vi "Check if Adjacent.vi"(8 "error in (no error)":errorcluster, 9 "Symbol.lvclass":refnum<class "Symbol.lvclass">, 10 "Number.lvclass":refnum<class "Number.lvclass">) -> (0 "error out":errorcluster, 2 "Is Adjacent?":bool)   [LabVIEW 2020, in "Schema Parser.lvclass"]
uses:
  Schema Parser.lvclass
  Number/Number.lvclass
  Symbol/Symbol.lvclass
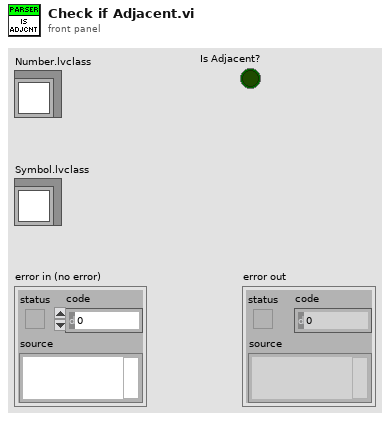
[diagram p1: front panel]
types:
  T1 = typedef "Symbol.lvclass/Coordinate.ctl" = cluster{"Col":i32, "Row":i32}
  T2 = typedef "Number.lvclass/Coordinate.ctl" = cluster{"Col":i32, "Row":i32}
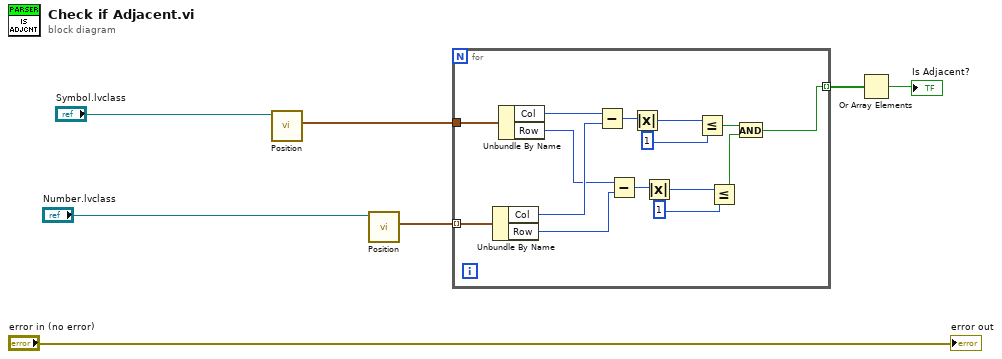
[diagram p0: block diagram]
diagram:
  n1 = call "Position.vi"("Number in"="Symbol.lvclass") -> ("Position"=w3:T1)  [unwired: 8 in, 2 out]
  n2 = call "Position.vi"("Number in"="Number.lvclass") -> ("Position"=w4:T2[])  [unwired: 8 in, 2 out]
  n3 = for {
    tunnel: w4 -> [w22] mode=indexing
    tunnel: w3 -> [w21]
    tunnel: [w9] -> w1 mode=indexing
    n4 = Unbundle By Name(w22) -> ("Col"=w19:i32, "Row"=w10:i32)
    n5 = Unbundle By Name(w21) -> ("Col"=w20:i32, "Row"=w11:i32)
    n6 = Subtract(x=w20, y=w19) -> (x-y=w18:i32)
    n7 = Subtract(x=w11, y=w10) -> (x-y=w12:i32)
    n8 = Absolute Value(x=w18) -> (abs(x)=w17:i32)
    n9 = Absolute Value(x=w12) -> (abs(x)=w13:i32)
    n10 = Less Or Equal?(x=w17, y=1) -> (x <= y?=w15:bool)
    n11 = Less Or Equal?(x=w13, y=1) -> (x <= y?=w8:bool)
    n12 = And(x=w15, y=w8) -> (x .and. y?=w9:bool)
  }
  n13 = Or Array Elements(Boolean array=w1) -> (logical OR=→"Is Adjacent?":bool)
  "error out" <- "error in (no error)"
